vi "SV TDMS Read.vi"   [LabVIEW 2017]
doc: "Reads the specified .tdms file and returns data in a format specific to the polymorphic instance selected."
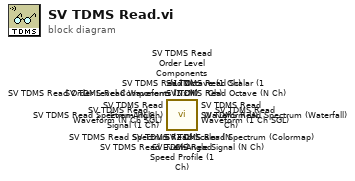
[diagram p0: block diagram]
diagram:
  n1 = call <vilib>:"SV TDMS Read Scalar (N Ch).vi"() -> ()  [unwired: 8 in, 8 out]
  n2 = call <vilib>:"SV TDMS Read Scalar (1 Ch).vi"() -> ()  [unwired: 8 in, 8 out]
  n3 = call <vilib>:"SV TDMS Read Waveform (N Ch SGL).vi"() -> ()  [unwired: 10 in, 6 out]
  n4 = call <vilib>:"SV TDMS Read Waveform (1 Ch SGL).vi"() -> ()  [unwired: 10 in, 6 out]
  n5 = call <vilib>:"SV TDMS Read Order Level Components (NxM).vi"() -> ()  [unwired: 9 in, 7 out]
  n6 = call <vilib>:"SV TDMS Read Order Level Components (1xM).vi"() -> ()  [unwired: 9 in, 7 out]
  n7 = call <vilib>:"SV TDMS Read Speed Profile (1 Ch).vi"() -> ()  [unwired: 9 in, 7 out]
  n8 = call <vilib>:"SV TDMS Read Spectrum (Colormap).vi"() -> ()  [unwired: 10 in, 6 out]
  n9 = call <vilib>:"SV TDMS Read Spectrum (Waterfall).vi"() -> ()  [unwired: 9 in, 7 out]
  n10 = call <vilib>:"SV TDMS Read Spectrum (N Ch).vi"() -> ()  [unwired: 9 in, 7 out]
  n11 = call <vilib>:"SV TDMS Read Spectrum (1 Ch).vi"() -> ()  [unwired: 9 in, 7 out]
  n12 = call <vilib>:"SV TDMS Read Octave (N Ch).vi"() -> ()  [unwired: 9 in, 7 out]
  n13 = call <vilib>:"SV TDMS Read Octave (1 Ch).vi"() -> ()  [unwired: 9 in, 7 out]
  n14 = call <vilib>:"SV TDMS Read Even-Angle Signal (N Ch).vi"() -> ()  [unwired: 9 in, 7 out]
  n15 = call <vilib>:"SV TDMS Read Even-Angle Signal (1 Ch).vi"() -> ()  [unwired: 9 in, 7 out]
  n16 = call <vilib>:"SV TDMS Read Waveform (N Ch).vi"() -> ()  [unwired: 10 in, 6 out]
  n17 = call <vilib>:"SV TDMS Read Waveform (1 Ch).vi"() -> ()  [unwired: 10 in, 6 out]
